vi "Set Audio Spectrum Notifier.vi"(8 "Error In":errorcluster, 10 "Audio Spectrum Notifier":refnum<notifier>, 11 "Audio Analyzer In":refnum<class "Audio Analyzer.lvclass">) -> (0 "Error Out":errorcluster, 3 "Audio Analyzer Out":refnum<class "Audio Analyzer.lvclass">)   [LabVIEW 2019, in "Audio Analyzer.lvclass"]
uses:
  Audio Analyzer.lvclass
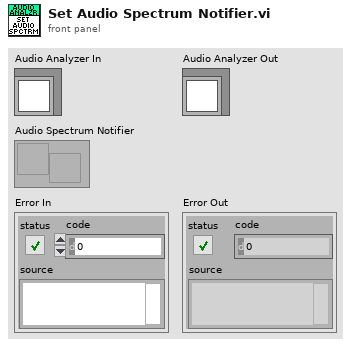
[diagram p1: front panel]
types:
  T1 = typedef "Audio Analyzer.lvclass/Data.ctl" = cluster{"Audio Spectrum Notifier":refnum<notifier>, "FPGA Reference":T2}
  T2 = typedef "Audio Analyzer.lvclass/FPGA Reference.ctl" = refnum<k20>
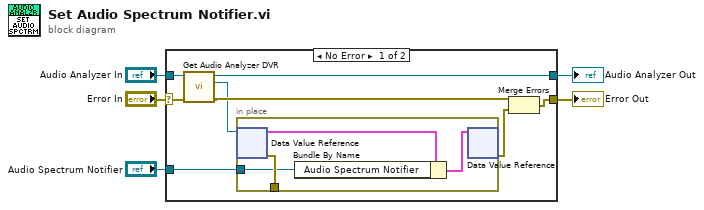
[diagram p0: block diagram]
diagram:
  n1 = case shown="No Error" "Error In" {
    selector: "Error In" -> [w9 w18]
    tunnel: [w12 w18] -> w2
    tunnel: [w8 w19] -> w5
    tunnel: "Audio Analyzer In" -> [w10 w19]
    tunnel: "Audio Spectrum Notifier" -> [w11 _]
    frame No Error {
      n2 = call "Get Audio Analyzer DVR.vi"("Error In"=w9, "Audio Analyzer In"=w10) -> ("Error Out"=w7:errorcluster, "DVR"=w6:refnum<data-value>, "Audio Analyzer Out"=w8:refnum<class "Audio Analyzer.lvclass">)  [unwired: 7 in]
      n3 = in-place {
        in-place-border: [w17] -> _
        in-place-border: w11 -> [w14]
        n4 = in-place-dvr #1(w6) -> (w16:T1, w17:errorcluster)
        n5 = Bundle By Name(cluster=w16, "Audio Spectrum Notifier"=w14) -> (w15:T1)
        n6 = in-place-dvr #1(w15) -> (w13:errorcluster)  [unwired: 1 out]
      }
      n7 = Merge Errors(w7, w13) -> (w12:errorcluster)
    }
    frame Error {
    }
  }
  "Audio Analyzer Out" <- w5
  "Error Out" <- w2
